vi "PH_PowerUnit_BaseClass.PU 2 Instancename.vi"(1 "PU":T1) -> (0 "Instance Name":string="N/A")   [LabVIEW 2014, in "PH_PowerUnit_BaseClass.lvlib"]
uses:
  PH_PowerUnit_BaseClass.lvlib
  PH_PP_Common/PH_PP_Common.PUs.ctl
  PH_PP_Common/PH_PP_Common.lvlib
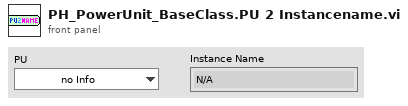
[diagram p1: front panel]
types:
  T1 = typedef "PH_PP_Common.lvlib/PH_PP_Common.PUs.ctl" = enum16{"no Info", "PA-19mm-1", "PA-19mm-2", "PA-45mm-PILC", "PA-45mm-MAIN", "MA-PU-1", "MA-PU-2", "MA-PU-3", "MA-PU-4", "MA-PU-5", "MA-PU-6", "MA-FR", "MA-PILC", "PA-45mm-DP"}
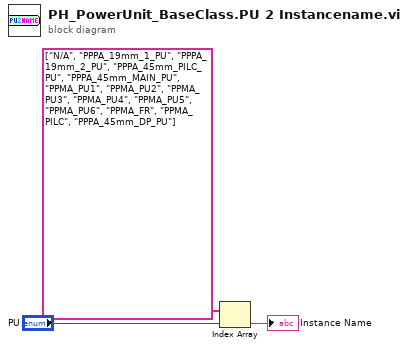
[diagram p0: block diagram]
diagram:
  n1 = Index Array(array=string[] ["N/A", "PPPA_19mm_1_PU", "PPPA_19mm_2_PU", "PPPA_45mm_PILC_PU", "PPPA_45mm_MAIN_PU", "PPMA_PU1", "PPMA_PU2", "PPMA_PU3", "PPMA_PU4", "PPMA_PU5", "PPMA_PU6", "PPMA_FR", "PPMA_PILC", "PPPA_45mm_DP_PU"], index="PU") -> (element=→"Instance Name":string)
